vi "NIYantraServer.vi"() -> ()   [LabVIEW 2012]
uses:
  <vilib>/userdefined/High Color/IMAQdx.ctl
  <vilib>/Instr/_visa.llb/VISA Configure Serial Port (Instr).vi
  <vilib>/Utility/file.llb/Write To Spreadsheet File (string).vi
  <vilib>/Utility/file.llb/Read From Spreadsheet File (string).vi
  <vilib>/Utility/file.llb/Read From Spreadsheet File (I64).vi
  <vilib>/vision/driver/NI_Vision_Acquisition_Software.lvlib
  <vilib>/vision/NI_Vision_Development_Module.lvlib
panel:
  out "Video":T1(plugin-control)
  out "Background":T1(plugin-control)
  out "Centroid":cluster{"X Centroid":sgl, "Y Centroid":sgl} {"Y Centroid" format="%.2f"; "X Centroid" format="%.2f"}
  out "No. of Particles":i32
  out "Binary Video":T1(plugin-control)
  in  "Threshold":cluster{"Lower value":sgl, "Upper value":sgl}={"Lower value"=50.255474, "Upper value"=255.0} {"Upper value" scale=0.0..255.0; "Lower value" scale=0.0..255.0}
  out "Centroid 1":cluster{"X Centroid":sgl, "Y Centroid":sgl} {"Y Centroid" format="%.2f"; "X Centroid" format="%.2f"}
  out "Final Centroid 1":sgl
  in  "Time Between Snaps (ms)":u32=500
  out "Centroid 2":cluster{"X Centroid":sgl, "Y Centroid":sgl} {"Y Centroid" format="%.2f"; "X Centroid" format="%.2f"}
  out "Final Centroid 2":sgl
  in  "Centroid Cutoff":dbl=130.0
  out "Bytes to be Written":i32
  out "Pedestrian":bool=TRUE
  out "Data Updated":bool=TRUE
  out "Output Array":string[](array[string])
  out "CAR":T2(ring)=enum."Do Not Write"
  out "Speed (Km/hr)":sgl
  in  "Wireless Address":u16(ring) items=["ab:cd:ef:gh:1", "ab:cd:ef:gh:2", "ab:cd:ef:gh:3", "ab:cd:ef:gh:4"]
  in  "Road Name":u16(ring)=1 items=["ISMD", "Bank More", "Jharia", "City Centre"]
  out "Fine Amount":dbl
  out "Total Fine":dbl
  out "Fine Imposed":dbl
  out "Fine Till Date":string
  out "Color":string
  out "Registration No.":string
  out "Car Name":string
  out "Wireless Owner":string
  out "Speed Limit":dbl
  out "Road Name":string
  out "Pedestrian Timer":dbl
  in  "Pedestrian\nTouch Button":bool
  out "Connection Status":bool
  out "Signal Timer":dbl
  out "Green2":bool
  out "Yellow2":bool
  out "Red2":bool=TRUE
  out "Over-Speed Alert":bool
  # "Inputs from the External Devices and Database"
  # "Examples"
  # "Car Details"
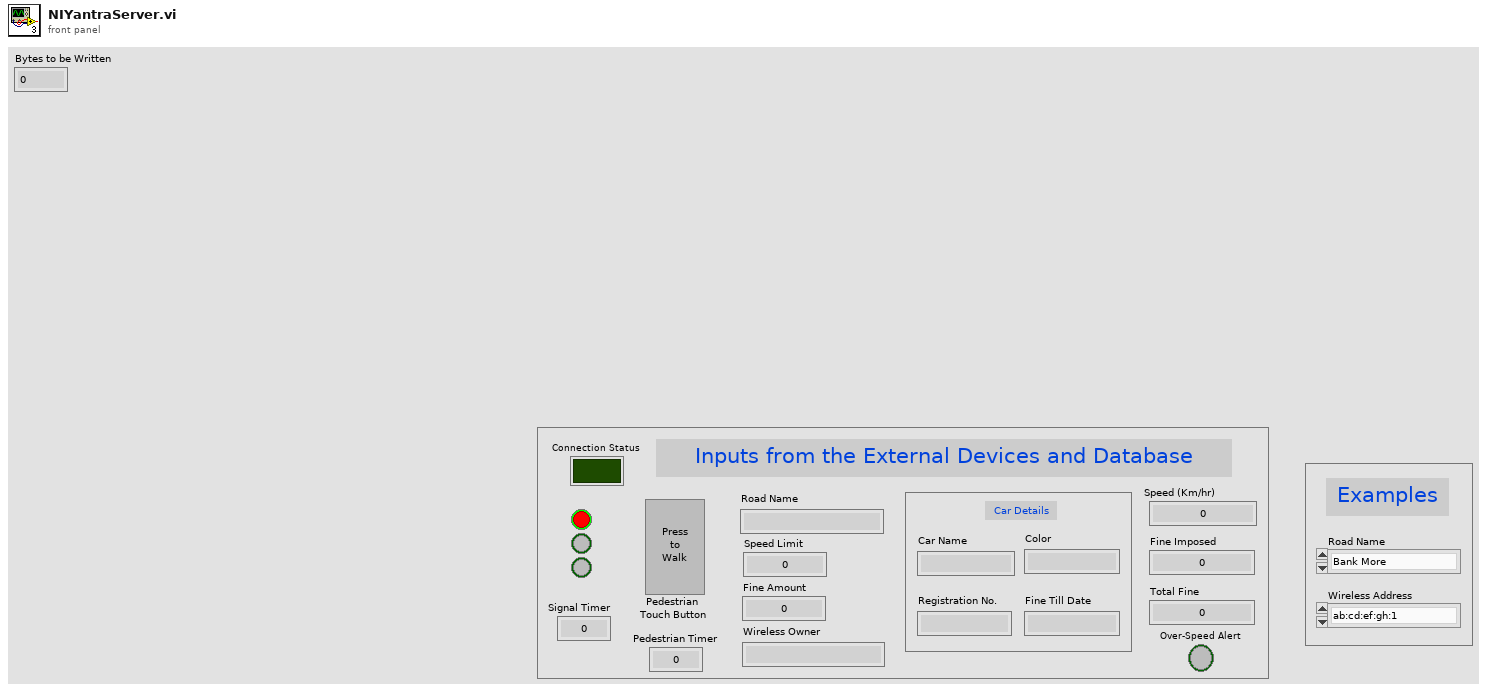
[diagram p1: front panel]
types:
  T1 = typedef "IMAQ Image.ctl" = refnum<image>
  T2 = enum16{"CAR1", "CAR2", "CAR3", "CAR4", "Do Not Write"}
  T3 = typedef "Image Type" = u32
  T4 = typedef "IMAQdx.ctl" = refnum<k21>
  T5 = cluster{"Red2":bool, "Yellow2":bool, "Green2":bool, "Signal Timer":dbl, "Pedestrian":bool, "Speed Limit":dbl, "Over-Speed Alert":bool, "Total Fine":dbl}
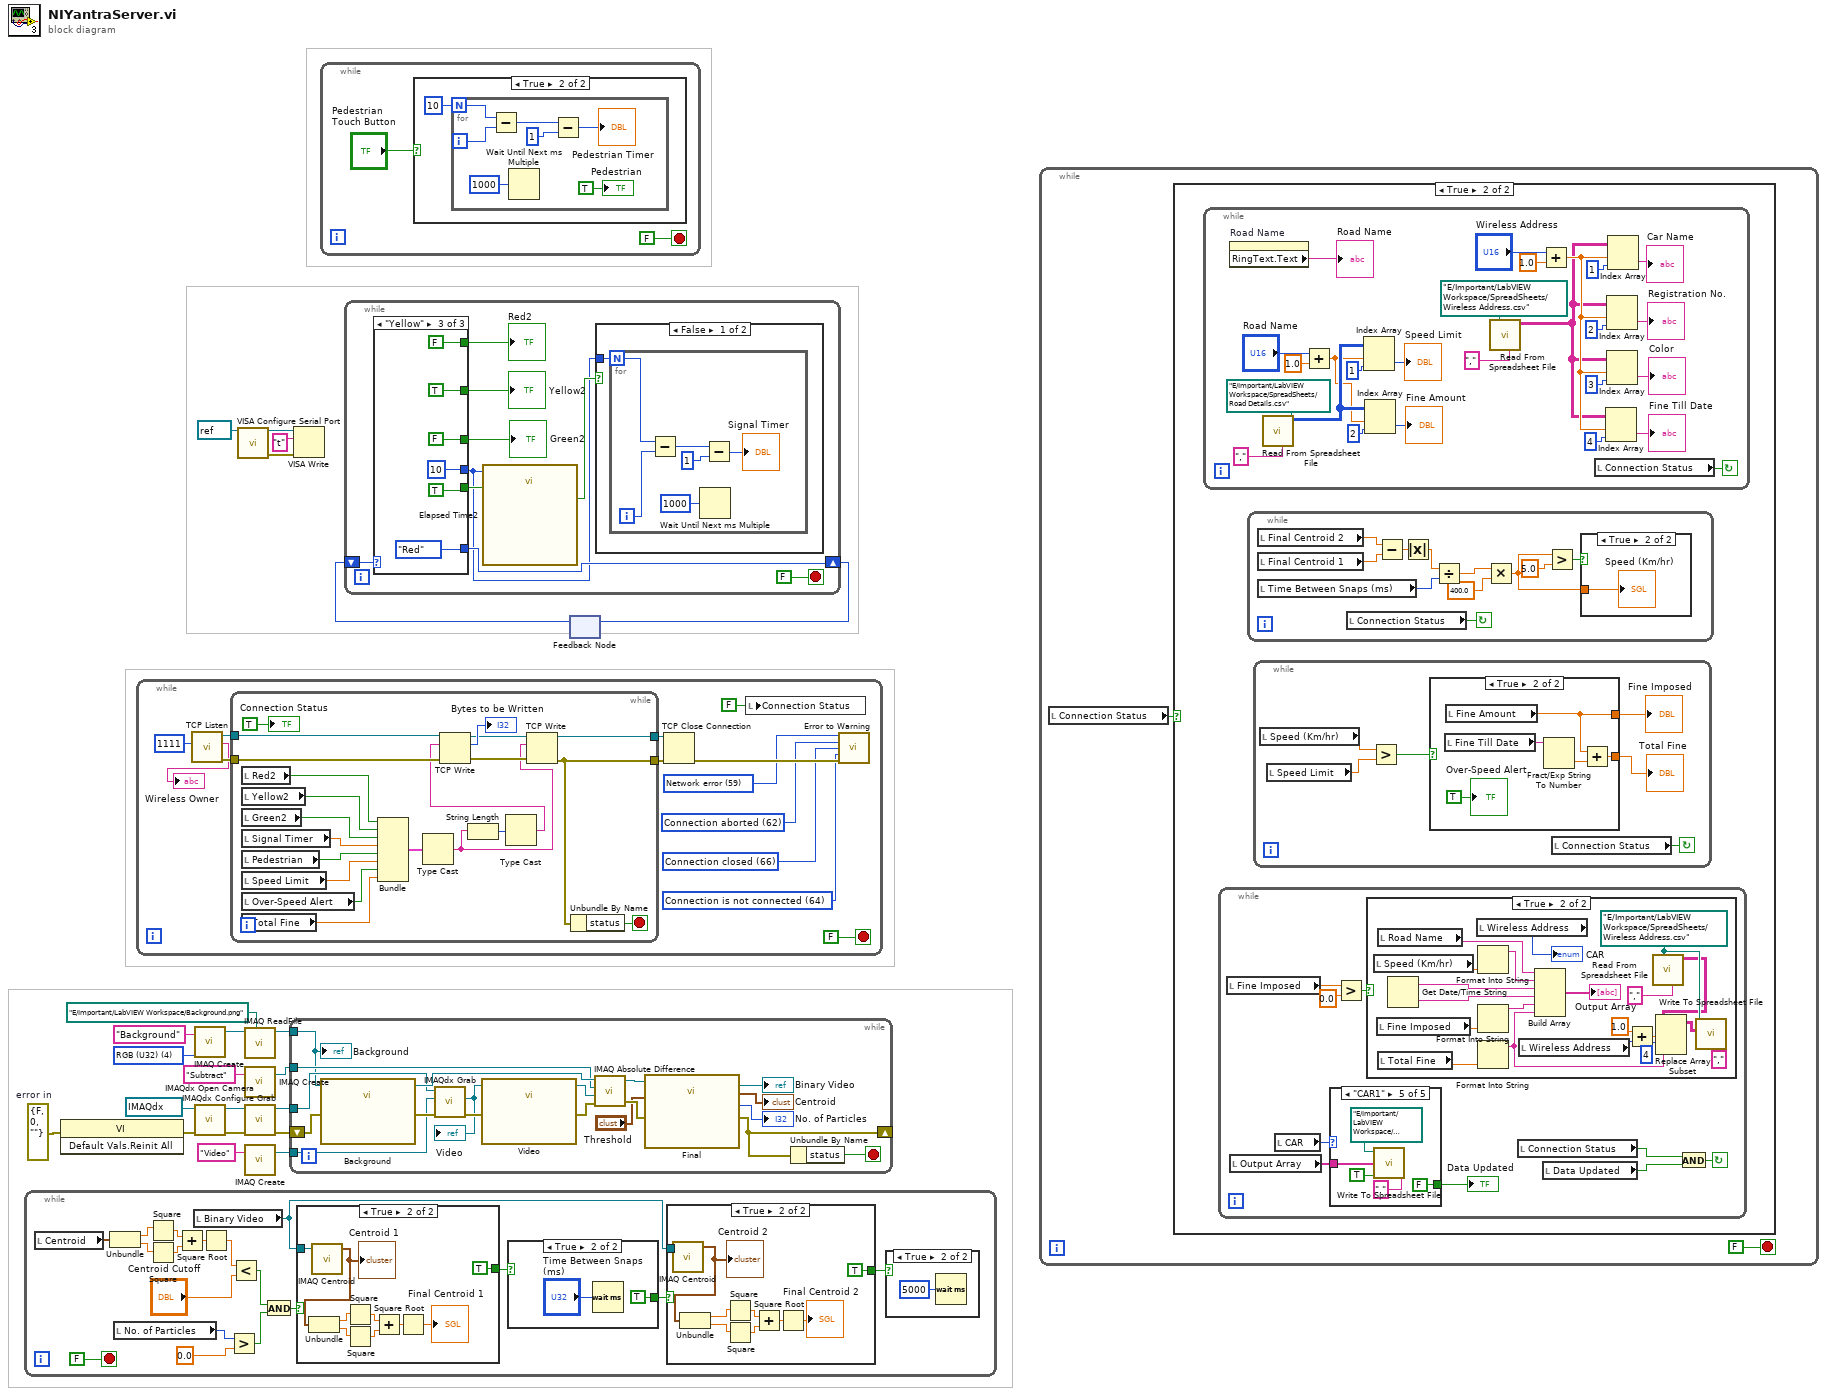
[diagram p0: block diagram]
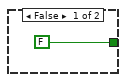
[diagram p3: hidden frame]
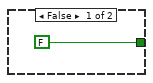
[diagram p4: hidden frame]
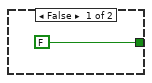
[diagram p5: hidden frame]
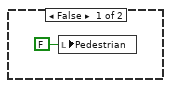
[diagram p6: hidden frame]
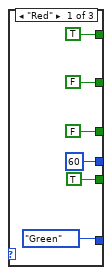
[diagram p8: hidden frame]
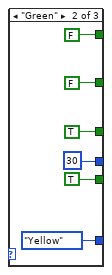
[diagram p9: hidden frame]
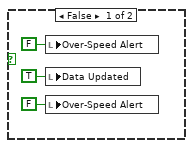
[diagram p10: hidden frame]
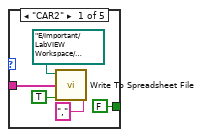
[diagram p11: hidden frame]
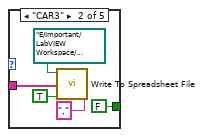
[diagram p12: hidden frame]
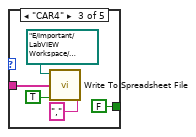
[diagram p13: hidden frame]
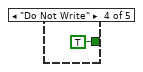
[diagram p14: hidden frame]
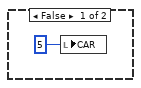
[diagram p15: hidden frame]
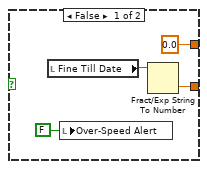
[diagram p17: hidden frame]
diagram:
  w9 = T3 4 items=["Grayscale (U8)", "Grayscale (I16)", "Grayscale (SGL)", "Complex (CSG)", "RGB (U32)", "HSL (U32)", "RGB (U64)", "Grayscale (U16)"] ("Image Type")
  w16 = errorcluster {"status"=FALSE, "code"=0, "source"=""}  # error in
  n1 = while {
    stop <- FALSE stop-if-true
    n2 = local read "Centroid"() -> (w40:cluster{"X Centroid":sgl, "Y Centroid":sgl})
    n3 = Unbundle(w40) -> ("X Centroid"=w33:sgl, "Y Centroid"=w28:sgl)
    n4 = local read "No. of Particles"() -> (w37:i32)
    n5 = Square(x=w33) -> (x^2=w30:sgl)
    n6 = Square(x=w28) -> (x^2=w31:sgl)
    n7 = Add(x=w30, y=w31) -> (x+y=w32:sgl)
    n8 = local read "Binary Video"() -> (w26:T1)
    n9 = Square Root(x=w32) -> (sqrt(x)=w27:sgl)
    n10 = Greater?(x=w37, y=0.0) -> (0:w35:bool)
    n11 = Less?(x=w27, y="Centroid Cutoff") -> (x < y?=w29:bool)
    n12 = And(x=w29, y=w35) -> (x .and. y?=w36:bool)
    n13 = case shown="True" w36 {
      tunnel: [FALSE TRUE] -> w25
      tunnel: w26 -> [_ w56]
      frame False {
      }
      frame True {
        n14 = call "IMAQ Centroid"("Image"=w56) -> ("Centroid"=w57:cluster{"X Centroid":sgl, "Y Centroid":sgl})  [unwired: 3 in, 1 out]
        "Centroid 1" <- w57
        n15 = Unbundle(w57) -> ("X Centroid"=w59:sgl, "Y Centroid"=w60:sgl)
        n16 = Square(x=w59) -> (x^2=w61:sgl)
        n17 = Square(x=w60) -> (x^2=w62:sgl)
        n18 = Add(x=w61, y=w62) -> (x+y=w63:sgl)
        n19 = Square Root(x=w63) -> (sqrt(x)=→"Final Centroid 1":sgl)
      }
    }
    n20 = case shown="True" w25 {
      tunnel: [FALSE TRUE] -> w24
      frame False {
      }
      frame True {
        n21 = Wait (ms)(milliseconds to wait="Time Between Snaps (ms)") -> ()  [unwired: 1 out]
      }
    }
    n22 = case shown="True" w24 {
      tunnel: w26 -> [_ w48]
      tunnel: [FALSE TRUE] -> w23
      frame False {
      }
      frame True {
        n23 = call "IMAQ Centroid"("Image"=w48) -> ("Centroid"=w47:cluster{"X Centroid":sgl, "Y Centroid":sgl})  [unwired: 3 in, 1 out]
        "Centroid 2" <- w47
        n24 = Unbundle(w47) -> ("X Centroid"=w50:sgl, "Y Centroid"=w51:sgl)
        n25 = Square(x=w50) -> (x^2=w52:sgl)
        n26 = Square(x=w51) -> (x^2=w53:sgl)
        n27 = Add(x=w52, y=w53) -> (x+y=w54:sgl)
        n28 = Square Root(x=w54) -> (sqrt(x)=→"Final Centroid 2":sgl)
      }
    }
    n29 = case shown="True" w23 {
      frame False {
      }
      frame True {
        n30 = Wait (ms)(milliseconds to wait=u32 5000) -> ()  [unwired: 1 out]
      }
    }
  }
  n31 = invoke class="VI" method="Default Vals.Reinit All"(error in=w16) -> (error out=w18:errorcluster)  [unwired: 2 in, 2 out]
  n32 = while {
    stop <- FALSE stop-if-true
    w69 = 62 items=["No Error", "Argument Error", "Memory Full", "Out of Zone", "End of File", "File Already Open", "Generic File IO Error", "File Not Found", "File Permission Error", "Disk Full", "Duplicate Path", "Too Many Files Open", "Not Enabled", "Resource File Not Found", "Cannot Add Resource", "Resource Not Found", "Image Not Found", "Image Memory Error", "Pen Does Not Exist", "Config Bad Type", "Config Token Not Found", "Config Parse Error", "Config Memory Error", "Bad External Code Format", "Bad External Code Offset", "External Code Not Present", "Null Window", "Destroy Window Mixup", "Null Menu", "Print Aborted", "Bad Print Record", "Print Driver Error", "Windows Error During Print", "Memory Error During Print", "Print Dialog Error", "Generic Print Error", "Invalid Device Refnum", "Device Not Found", "Device Parameter Error", "Device Unit Error", "Can't Open Device", "Device Call Aborted", "Generic Error", "Cancelled By User", "Object ID Too Low", "Object ID Too High", "Object Not In Heap", "Unknown Heap", "Bad DefProc ID", "DefProc Not In Table", "Message Out Of Range", "Null Method", "Unknown Message", "Manager Call Not Supported", "Bad address", "Connection In progress", "Connection timed out", "Connection is already in progress", "Network attribute not supported", "Network error", "Address in use", "System out of memory", "Connection aborted", "Connection refused", "Connection is not connected", "Connection is already connected", "Connection closed", "Initialize error (interapplication manager)", "Bad occurrence", "Wait on unbound occurrence handler", "Occurrence queue overflow", "Bad path", "Semaphore not signaled", "Unrecognized type (interapplication manager)"] ("4th Error to Convert")
    w67 = 64 items=["No Error", "Argument Error", "Memory Full", "Out of Zone", "End of File", "File Already Open", "Generic File IO Error", "File Not Found", "File Permission Error", "Disk Full", "Duplicate Path", "Too Many Files Open", "Not Enabled", "Resource File Not Found", "Cannot Add Resource", "Resource Not Found", "Image Not Found", "Image Memory Error", "Pen Does Not Exist", "Config Bad Type", "Config Token Not Found", "Config Parse Error", "Config Memory Error", "Bad External Code Format", "Bad External Code Offset", "External Code Not Present", "Null Window", "Destroy Window Mixup", "Null Menu", "Print Aborted", "Bad Print Record", "Print Driver Error", "Windows Error During Print", "Memory Error During Print", "Print Dialog Error", "Generic Print Error", "Invalid Device Refnum", "Device Not Found", "Device Parameter Error", "Device Unit Error", "Can't Open Device", "Device Call Aborted", "Generic Error", "Cancelled By User", "Object ID Too Low", "Object ID Too High", "Object Not In Heap", "Unknown Heap", "Bad DefProc ID", "DefProc Not In Table", "Message Out Of Range", "Null Method", "Unknown Message", "Manager Call Not Supported", "Bad address", "Connection In progress", "Connection timed out", "Connection is already in progress", "Network attribute not supported", "Network error", "Address in use", "System out of memory", "Connection aborted", "Connection refused", "Connection is not connected", "Connection is already connected", "Connection closed", "Initialize error (interapplication manager)", "Bad occurrence", "Wait on unbound occurrence handler", "Occurrence queue overflow", "Bad path", "Semaphore not signaled", "Unrecognized type (interapplication manager)"] ("3rd Error to Convert")
    w68 = 66 items=["No Error", "Argument Error", "Memory Full", "Out of Zone", "End of File", "File Already Open", "Generic File IO Error", "File Not Found", "File Permission Error", "Disk Full", "Duplicate Path", "Too Many Files Open", "Not Enabled", "Resource File Not Found", "Cannot Add Resource", "Resource Not Found", "Image Not Found", "Image Memory Error", "Pen Does Not Exist", "Config Bad Type", "Config Token Not Found", "Config Parse Error", "Config Memory Error", "Bad External Code Format", "Bad External Code Offset", "External Code Not Present", "Null Window", "Destroy Window Mixup", "Null Menu", "Print Aborted", "Bad Print Record", "Print Driver Error", "Windows Error During Print", "Memory Error During Print", "Print Dialog Error", "Generic Print Error", "Invalid Device Refnum", "Device Not Found", "Device Parameter Error", "Device Unit Error", "Can't Open Device", "Device Call Aborted", "Generic Error", "Cancelled By User", "Object ID Too Low", "Object ID Too High", "Object Not In Heap", "Unknown Heap", "Bad DefProc ID", "DefProc Not In Table", "Message Out Of Range", "Null Method", "Unknown Message", "Manager Call Not Supported", "Bad address", "Connection In progress", "Connection timed out", "Connection is already in progress", "Network attribute not supported", "Network error", "Address in use", "System out of memory", "Connection aborted", "Connection refused", "Connection is not connected", "Connection is already connected", "Connection closed", "Initialize error (interapplication manager)", "Bad occurrence", "Wait on unbound occurrence handler", "Occurrence queue overflow", "Bad path", "Semaphore not signaled", "Unrecognized type (interapplication manager)"] ("2nd Error to Convert")
    w70 = 59 items=["No Error", "Argument Error", "Memory Full", "Out of Zone", "End of File", "File Already Open", "Generic File IO Error", "File Not Found", "File Permission Error", "Disk Full", "Duplicate Path", "Too Many Files Open", "Not Enabled", "Resource File Not Found", "Cannot Add Resource", "Resource Not Found", "Image Not Found", "Image Memory Error", "Pen Does Not Exist", "Config Bad Type", "Config Token Not Found", "Config Parse Error", "Config Memory Error", "Bad External Code Format", "Bad External Code Offset", "External Code Not Present", "Null Window", "Destroy Window Mixup", "Null Menu", "Print Aborted", "Bad Print Record", "Print Driver Error", "Windows Error During Print", "Memory Error During Print", "Print Dialog Error", "Generic Print Error", "Invalid Device Refnum", "Device Not Found", "Device Parameter Error", "Device Unit Error", "Can't Open Device", "Device Call Aborted", "Generic Error", "Cancelled By User", "Object ID Too Low", "Object ID Too High", "Object Not In Heap", "Unknown Heap", "Bad DefProc ID", "DefProc Not In Table", "Message Out Of Range", "Null Method", "Unknown Message", "Manager Call Not Supported", "Bad address", "Connection In progress", "Connection timed out", "Connection is already in progress", "Network attribute not supported", "Network error", "Address in use", "System out of memory", "Connection aborted", "Connection refused", "Connection is not connected", "Connection is already connected", "Connection closed", "Initialize error (interapplication manager)", "Bad occurrence", "Wait on unbound occurrence handler", "Occurrence queue overflow", "Bad path", "Semaphore not signaled", "Unrecognized type (interapplication manager)"] ("1st Error to Convert")
    n33 = call <vilib>:"TCP Listen.vi"("port"=u16 1111) -> ("error out"=w75:errorcluster, "remote address"=→"Wireless Owner":string, "connection ID"=w76:refnum<k5>)  [unwired: 6 in, 2 out]
    n34 = while {
      tunnel: w76 -> [w95]
      tunnel: w75 -> [w94]
      tunnel: [w79] -> w72
      tunnel: [w96] -> w71
      stop <- w98 stop-if-true
      n35 = local read "Red2"() -> (w90:bool)
      n36 = local read "Yellow2"() -> (w89:bool)
      n37 = local read "Green2"() -> (w88:bool)
      n38 = local read "Signal Timer"() -> (w87:dbl)
      n39 = local read "Pedestrian"() -> (w86:bool)
      n40 = local read "Speed Limit"() -> (w85:dbl)
      n41 = local read "Over-Speed Alert"() -> (w84:bool)
      n42 = local read "Total Fine"() -> (w83:dbl)
      n43 = Bundle("Red2"=w90, "Yellow2"=w89, "Green2"=w88, "Signal Timer"=w87, "Pedestrian"=w86, "Speed Limit"=w85, "Over-Speed Alert"=w84, "Total Fine"=w83) -> (w97:T5)  [unwired: 1 in]
      n44 = Type Cast(x=w97) -> (*(type *) &x=w80:string)  [unwired: 1 in]
      n45 = String Length(string=w80) -> (length=w82:i32)
      n46 = Type Cast(x=w82) -> (*(type *) &x=w81:string)  [unwired: 1 in]
      n47 = TCP Write(connection ID=w95, data in=w81, error in (no error)=w94) -> (connection ID out=w92:refnum<k5>, bytes written=→"Bytes to be Written":i32, error out=w91:errorcluster)  [unwired: 1 in]
      n48 = TCP Write(connection ID=w92, data in=w80, error in (no error)=w91) -> (connection ID out=w96:refnum<k5>, error out=w79:errorcluster)  [unwired: 1 in, 1 out]
      n49 = Unbundle By Name(w79) -> ("status"=w98:bool)
      "Connection Status" <- TRUE ("Connection Status")
    }
    n50 = TCP Close Connection(connection ID=w71, error in (no error)=w72) -> (error out=w74:errorcluster)  [unwired: 1 in, 1 out]
    n51 = local write "Connection Status"(FALSE ("Connection Status")) -> ()
    n52 = call <vilib>:"Error to Warning.vi"("1st Error to Convert"=w70, "2nd Error to Convert"=w69, "3rd Error to Convert"=w68, "4th Error to Convert"=w67, "error in"=w74) -> ()  [unwired: 11 out]
  }
  n53 = call "IMAQ Create"("Image Name"="Background", "Image Type"=w9) -> ("New Image"=w8:T1)  [unwired: 3 in, 1 out]
  n54 = call <vilib>:"IMAQdx Open Camera.vi"("error in"=w18, "Session In"=T4 "cam0") -> ("error out"=w17:errorcluster, "Session Out"=w20:T4)  [unwired: 8 in]
  n55 = call-poly "VISA Configure Serial Port"("VISA resource name"=refnum<visa-resource-name> refnum) -> ("VISA resource name out"=w3:refnum<visa-resource-name>, "error out"=w2:errorcluster)  [unwired: 13 in]
  n56 = call "IMAQ ReadFile"("File Path"=path "E:/Important/LabVIEW Workspace/Background.png", "Image"=w8) -> ("Image Out"=w7:T1)  [unwired: 5 in, 4 out]
  n57 = call "IMAQ Create"("Image Name"="Subtract") -> ("New Image"=w11:T1)  [unwired: 4 in, 1 out]
  n58 = call <vilib>:"IMAQdx Configure Grab.vi"("error in"=w17, "Session In"=w20) -> ("error out"=w14:errorcluster, "Session Out"=w15:T4)  [unwired: 8 in]
  n59 = call "IMAQ Create"("Image Name"="Video") -> ("New Image"=w5:T1)  [unwired: 4 in, 1 out]
  n60 = while {
    tunnel: w15 -> [w101]
    tunnel: w11 -> [w102]
    shift-right: [w104] -> _
    shift-left: w14 -> [w103]
    tunnel: w7 -> [w100]
    tunnel: w5 -> [w99]
    stop <- w117 stop-if-true
    n61 = call "Background"("Image In"=w100, "error in"=w103) -> ("Image Out"=w109:T1, "error out"=w115:errorcluster)  [unwired: 24 in]
    n62 = call <vilib>:"IMAQdx Grab.vi"("error in"=w115, "Image In"=w99, "Session In"=w101) -> ("error out"=w114:errorcluster, "Image Out"=w105:T1)  [unwired: 5 in, 2 out]
    "Video" <- w105
    n63 = call "Video"("Image In"=w105, "error in"=w114) -> ("Image Out"=w116:T1, "error out"=w113:errorcluster)  [unwired: 24 in]
    n64 = call "IMAQ Absolute Difference"("Image Src A"=w109, "Image Dst"=w102, "Image Src B"=w116, "error in (no error)"=w113) -> ("Image Dst Out"=w112:T1, "error out"=w111:errorcluster)  [unwired: 3 in]
    n65 = call "Final"("Image In"=w112, "Range (Threshold Set)"="Threshold", "error in"=w111) -> ("Image Out"=→"Binary Video":T1, "Centroid (Centroid)"=→"Centroid":cluster{"X Centroid":sgl, "Y Centroid":sgl}, "Number of Particles (Particle Analysis)"=→"No. of Particles":i32, "error out"=w104:errorcluster)  [unwired: 21 in]
    n66 = Unbundle By Name(w104) -> ("status"=w117:bool)
    "Background" <- w100
  }
  n67 = VISA Write(VISA resource name=w3, write buffer="t", error in (no error)=w2) -> ()  [unwired: 3 out]
  n68 = while {
    stop <- FALSE stop-if-true
    n69 = case shown="True" "Pedestrian\nTouch Button" {
      frame False {
        n70 = local write "Pedestrian"(FALSE ("Pedestrian")) -> ()
      }
      frame True {
        n71 = for {
          N: 10 -> [w128]
          i -> [w127]
          n72 = Subtract(x=w128, y=w127) -> (x-y=w125:i32)
          n73 = Wait Until Next ms Multiple(millisecond multiple=u32 1000) -> ()  [unwired: 1 out]
          n74 = Subtract(x=w125, y=1) -> (x-y=→"Pedestrian Timer":i32)
          "Pedestrian" <- TRUE ("Boolean")
        }
      }
    }
  }
  n75 = feedback #1() -> (w21:enum16{"Red", "Yellow", "Green"})  [unwired: 1 in]
  n76 = while {
    shift-right: [w133] -> w22
    shift-left: w21 -> [w134]
    stop <- FALSE stop-if-true
    n77 = case shown="\"Yellow\"" w134 {
      tunnel: [TRUE FALSE FALSE] -> w137
      tunnel: [FALSE FALSE TRUE] -> w136
      tunnel: [FALSE TRUE FALSE] -> w135
      tunnel: [enum16{"Red", "Yellow", "Green"}."Green" enum16{"Red", "Yellow", "Green"}."Yellow" enum16{"Red", "Yellow", "Green"}."Red"] -> w133
      tunnel: [TRUE ("Reset") TRUE ("Reset") TRUE ("Reset")] -> w132
      tunnel: [60 ("x") 30 ("x") 10 ("x")] -> w130
      frame "Red" {
      }
      frame "Green" {
      }
      frame "Yellow" {
      }
    }
    "Red2" <- w137
    "Yellow2" <- w136
    "Green2" <- w135
    n78 = call "Elapsed Time2"("Time Target (s)"=w130, "Reset"=w132) -> ("Time has Elapsed"=w131:bool)  [unwired: 10 in, 7 out]
    n79 = case shown="False" w131 {
      tunnel: w130 -> [w138 _]
      frame False {
        n80 = for {
          N: w138 -> [w142]
          i -> [w143]
          n81 = Subtract(x=w142, y=w143) -> (x-y=w141:i32)
          n82 = Wait Until Next ms Multiple(millisecond multiple=u32 1000) -> ()  [unwired: 1 out]
          n83 = Subtract(x=w141, y=1) -> (x-y=→"Signal Timer":i32)
        }
      }
      frame True {
      }
    }
  }
  n84 = feedback-in #1(w22) -> ()
  n85 = while {
    stop <- FALSE stop-if-true
    n86 = local read "Connection Status"() -> (w163:bool)
    n87 = case shown="True" w163 {
      frame False {
        n88 = local write "Over-Speed Alert"(FALSE ("Over-Speed Alert")) -> ()
        n89 = local write "Data Updated"(TRUE ("Data Updated")) -> ()
        n90 = local write "Over-Speed Alert"(FALSE ("Over-Speed Alert")) -> ()
      }
      frame True {
        n91 = while {
          stop <- w247 continue-if-true
          n92 = property on="Road Name" class="Ring (strict)"() -> ("RingText.Text"=→"Road Name":string)  [unwired: 2 in, 2 out]
          n93 = call-poly <vilib>:"Read From Spreadsheet File.vi"("delimiter (\\t)"="," ("delimiter (\\t)"), "file path (dialog if empty)"=path "E:/Important/LabVIEW Workspace/SpreadSheets/Road Details.csv") -> ("all rows"=w259:i64[][])  [unwired: 5 in, 4 out]
          n94 = Add(x="Road Name", y=1.0) -> (x+y=w258:dbl)
          n95 = Index Array(array=w259, index (row)=w258, index (col)=1 ("disabled index (col)")) -> (element=→"Speed Limit":i64)
          n96 = Index Array(array=w259, index (row)=w258, index (col)=2 ("disabled index (col)")) -> (element=→"Fine Amount":i64)
          n97 = call-poly <vilib>:"Read From Spreadsheet File.vi"("delimiter (\\t)"="," ("delimiter (\\t)"), "file path (dialog if empty)"=path "E:/Important/LabVIEW Workspace/SpreadSheets/Wireless Address.csv") -> ("all rows"=w248:string[][])  [unwired: 5 in, 4 out]
          n98 = Add(x="Wireless Address", y=1.0) -> (x+y=w249:dbl)
          n99 = local read "Connection Status"() -> (w247:bool)
          n100 = Index Array(array=w248, index (row)=w249, index (col)=4 ("disabled index (col)")) -> (element=→"Fine Till Date":string)
          n101 = Index Array(array=w248, index (row)=w249, index (col)=2 ("disabled index (col)")) -> (element=→"Registration No.":string)
          n102 = Index Array(array=w248, index (row)=w249, index (col)=3 ("disabled index (col)")) -> (element=→"Color":string)
          n103 = Index Array(array=w248, index (row)=w249, index (col)=1 ("disabled index (col)")) -> (element=→"Car Name":string)
        }
        n104 = while {
          stop <- w171 continue-if-true
          n105 = local read "Fine Imposed"() -> (w176:dbl)
          n106 = local read "Output Array"() -> (w169:string[])
          n107 = local read "CAR"() -> (w170:T2)
          n108 = case shown="\"CAR1\"" w170 {
            tunnel: w169 -> [w178 w183 w188 _ w194]
            tunnel: [FALSE ("append to file? (new file:F)") FALSE ("append to file? (new file:F)") FALSE ("append to file? (new file:F)") TRUE ("append to file? (new file:F)") FALSE ("append to file? (new file:F)")] -> w168
            frame "CAR2" {
              n109 = call-poly <vilib>:"Write To Spreadsheet File.vi"("delimiter (\\t)"="," ("delimiter (\\t)"), "append to file? (new file:F)"=TRUE, "1D data"=w178, "file path (dialog if empty)"=path "E:/Important/LabVIEW Workspace/SpreadSheets/CAR2.csv") -> ()  [unwired: 4 in, 1 out]
            }
            frame "CAR3" {
              n110 = call-poly <vilib>:"Write To Spreadsheet File.vi"("delimiter (\\t)"="," ("delimiter (\\t)"), "append to file? (new file:F)"=TRUE, "1D data"=w183, "file path (dialog if empty)"=path "E:/Important/LabVIEW Workspace/SpreadSheets/CAR3.csv") -> ()  [unwired: 4 in, 1 out]
            }
            frame "CAR4" {
              n111 = call-poly <vilib>:"Write To Spreadsheet File.vi"("delimiter (\\t)"="," ("delimiter (\\t)"), "append to file? (new file:F)"=TRUE, "1D data"=w188, "file path (dialog if empty)"=path "E:/Important/LabVIEW Workspace/SpreadSheets/CAR4.csv") -> ()  [unwired: 4 in, 1 out]
            }
            frame "Do Not Write" {
            }
            frame "CAR1" {
              n112 = call-poly <vilib>:"Write To Spreadsheet File.vi"("delimiter (\\t)"="," ("delimiter (\\t)"), "append to file? (new file:F)"=TRUE, "1D data"=w194, "file path (dialog if empty)"=path "E:/Important/LabVIEW Workspace/SpreadSheets/CAR1.csv") -> ()  [unwired: 4 in, 1 out]
            }
          }
          "Data Updated" <- w168
          n113 = Greater?(x=w176, y=0.0) -> (0:w174:bool)
          n114 = case shown="True" w174 {
            frame False {
              n115 = local write "CAR"(u32 5 ("milliseconds to wait")) -> ()
            }
            frame True {
              w205 = path "E:/Important/LabVIEW Workspace/SpreadSheets/Wireless Address.csv" ("file path (dialog if empty)")
              n116 = local read "Speed (Km/hr)"() -> (w210:sgl)
              n117 = local read "Fine Imposed"() -> (w211:dbl)
              n118 = local read "Road Name"() -> (w214:string)
              n119 = local read "Total Fine"() -> (w213:dbl)
              n120 = Get Date/Time String() -> (date string=w216:string, time string=w217:string)  [unwired: 3 in]
              n121 = local read "Wireless Address"() -> (→"CAR":u16)
              n122 = Format Into String(w210) -> (resulting string=w215:string)  [unwired: 3 in, 1 out]
              n123 = Format Into String(w211) -> (resulting string=w212:string)  [unwired: 3 in, 1 out]
              n124 = Format Into String(w213) -> (resulting string=w209:string)  [unwired: 3 in, 1 out]
              n125 = local read "Wireless Address"() -> (w200:u16)
              n126 = Build Array(w214, w215, w216, w217, w212, w209) -> (→"Output Array":string[])
              n127 = Add(x=1.0 ("y"), y=w200) -> (x+y=w202:dbl)
              n128 = call-poly <vilib>:"Read From Spreadsheet File.vi"("delimiter (\\t)"="," ("delimiter (\\t)"), "file path (dialog if empty)"=w205) -> ("all rows"=w203:string[][])  [unwired: 5 in, 4 out]
              n129 = Replace Array Subset(array=w203, new element=w209, index (row)=w202, index (col)=4 ("disabled index (col)")) -> (w207:string[][])
              n130 = call-poly <vilib>:"Write To Spreadsheet File.vi"("delimiter (\\t)"="," ("delimiter (\\t)"), "2D data"=w207, "file path (dialog if empty)"=w205) -> ()  [unwired: 5 in, 1 out]
            }
          }
          n131 = local read "Connection Status"() -> (w173:bool)
          n132 = local read "Data Updated"() -> (w172:bool)
          n133 = And(x=w173, y=w172) -> (x .and. y?=w171:bool)
        }
        n134 = while {
          stop <- w229 continue-if-true
          n135 = local read "Final Centroid 2"() -> (w219:sgl)
          n136 = local read "Final Centroid 1"() -> (w220:sgl)
          n137 = local read "Time Between Snaps (ms)"() -> (w223:u32)
          n138 = local read "Connection Status"() -> (w229:bool)
          n139 = Subtract(x=w219, y=w220) -> (x-y=w221:sgl)
          n140 = Absolute Value(x=w221) -> (abs(x)=w222:sgl)
          n141 = Divide(x=w222, y=w223) -> (x/y=w224:sgl)
          n142 = Multiply(x=w224, y=sgl 400.0) -> (x*y=w227:sgl)
          n143 = Greater?(x=w227, y=5.0) -> (0:w228:bool)
          n144 = case shown="True" w228 {
            tunnel: w227 -> [_ w230]
            frame False {
            }
            frame True {
              "Speed (Km/hr)" <- w230
            }
          }
        }
        n145 = while {
          stop <- w234 continue-if-true
          n146 = local read "Speed (Km/hr)"() -> (w236:sgl)
          n147 = local read "Speed Limit"() -> (w235:dbl)
          n148 = Greater?(x=w236, y=w235) -> (0:w233:bool)
          n149 = case shown="True" w233 {
            tunnel: [w239 w242] -> w232
            tunnel: [0.0 ("Fine Amount") w241] -> w231
            frame False {
              n150 = local read "Fine Till Date"() -> (w238:string)
              n151 = local write "Over-Speed Alert"(FALSE ("Over-Speed Alert")) -> ()
              n152 = Fract/Exp String To Number(string=w238) -> (number=w239:dbl)  [unwired: 3 in, 1 out]
            }
            frame True {
              n153 = local read "Fine Till Date"() -> (w244:string)
              n154 = local read "Fine Amount"() -> (w241:dbl)
              n155 = Fract/Exp String To Number(string=w244) -> (number=w243:dbl)  [unwired: 3 in, 1 out]
              n156 = Add(x=w241, y=w243) -> (x+y=w242:dbl)
              "Over-Speed Alert" <- TRUE ("Over-Speed Alert")
            }
          }
          "Total Fine" <- w232
          "Fine Imposed" <- w231
          n157 = local read "Connection Status"() -> (w234:bool)
        }
      }
    }
  }
